vi "Esercitazione 6 - Elementi comuni Array.vi"() -> ()   [LabVIEW 2018]
panel:
  out "Array 3":dbl[][](array[numeric])
  in  "Array 2":dbl[](array[numeric])
  in  "Array":dbl[](array[numeric])
  # "restituire un array (C)\nche contenga soltanto\ni valori numerici presenti\nsia in (A) che in (B)"
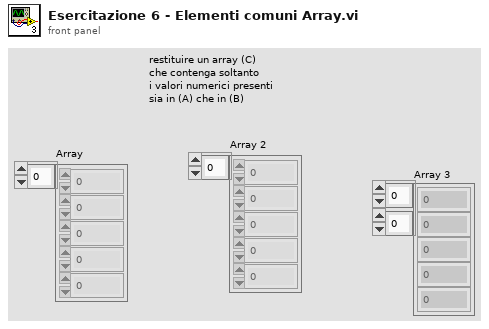
[diagram p1: front panel]
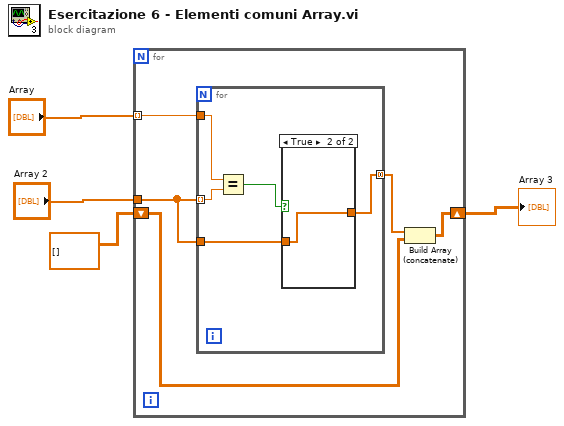
[diagram p0: block diagram]
diagram:
  n1 = for {
    tunnel: "Array" -> [w9] mode=indexing
    tunnel: "Array 2" -> [w7]
    shift-right: [w6] -> w1
    shift-left: dbl[][] [] -> [w5]
    n2 = for {
      tunnel: w9 -> [w12]
      tunnel: w7 -> [w14] mode=indexing
      tunnel: [w10] -> w8 mode=concatenating
      tunnel: w7 -> [w11]
      n3 = Equal?(x=w12, y=w14) -> (x = y?=w13:bool)
      n4 = case shown="True" w13 {
        tunnel: w11 -> [_ w15]
        tunnel: [_ w15] -> w10
        frame False {
        }
        frame True {
        }
      }
    }
    n5 = Build Array (concatenate)(w8, w5) -> (w6:dbl[][])
  }
  "Array 3" <- w1
